vi "Queue Out.vi"(8 "error in (no error)":errorcluster caption="Error In", 10 "Monitor":string, 11 "Queue In":refnum<queue>) -> (0 "error out":errorcluster caption="Error Out", 1 "Data":variant, 2 "Message":string, 3 "Queue Out":refnum<queue>, 4 "Queue NUmber":i32)   [LabVIEW 2020]
uses:
  Queue Message.ctl
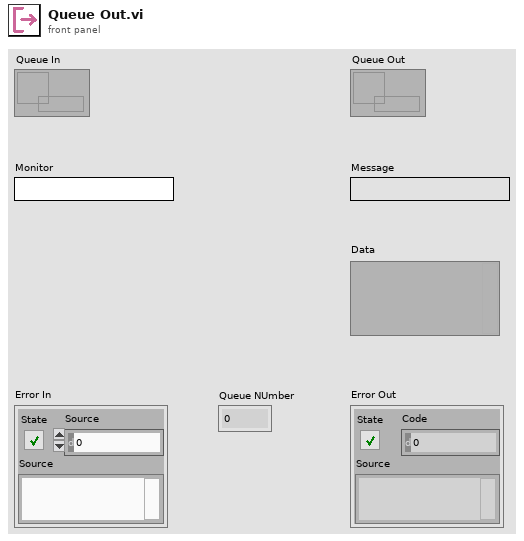
[diagram p1: front panel]
types:
  T1 = typedef "Queue Message.ctl" = cluster{"Message":string, "Data":variant}
  T2 = cluster{"Time":string, "Name":string, "Message":string, "Data":variant, "elements":i32}
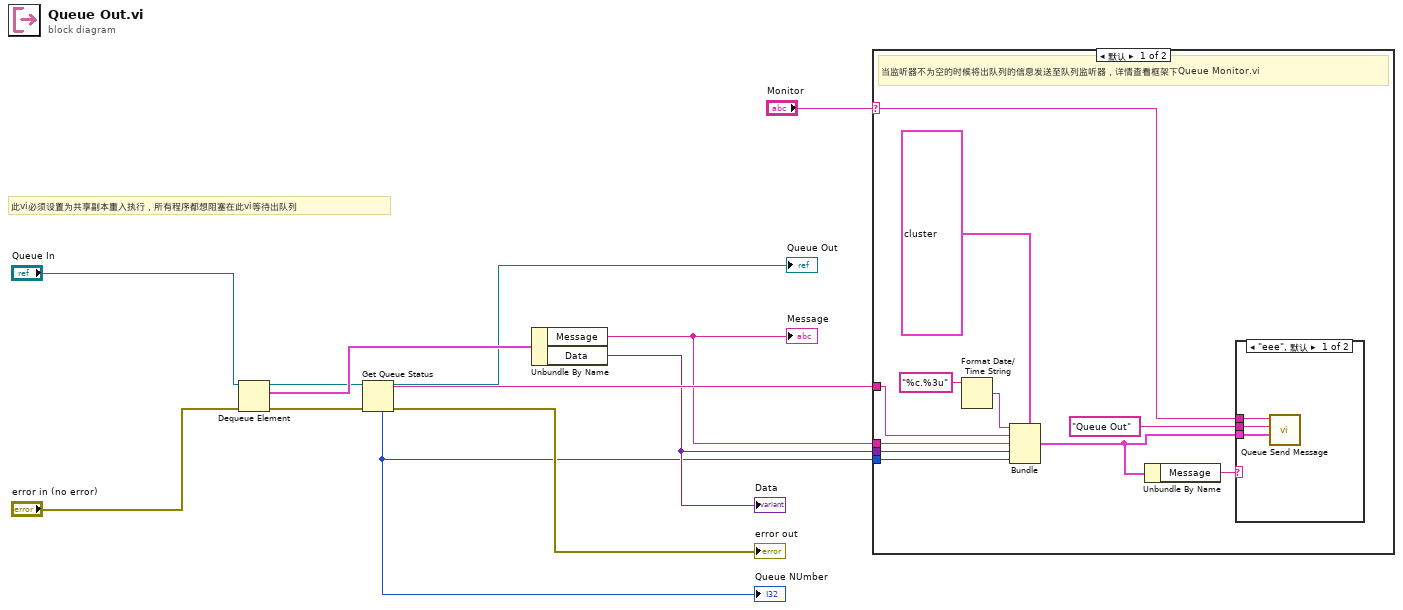
[diagram p0: block diagram]
diagram:
  # "此vi必须设置为共享副本重入执行，所有程序都想阻塞在此vi等待出队列"
  n1 = Dequeue Element(queue="Queue In", error in (no error)="error in (no error)") -> (queue out=w9:refnum<queue>, element=w11:T1, error out=w8:errorcluster)  [unwired: 1 in, 1 out]
  n2 = Get Queue Status(queue=w9, error in (no error)=w8) -> (queue out=→"Queue Out":refnum<queue>, queue name=w4:string, error out=→"error out":errorcluster, # elements in queue=w1:i32)  [unwired: 1 in, 4 out]
  "Queue NUmber" <- w1
  n3 = Unbundle By Name(w11) -> ("Message"=w3:string, "Data"=w2:variant)
  "Message" <- w3
  "Data" <- w2
  n4 = case shown="默认" "Monitor" {
    selector: "Monitor" -> [w23 _]
    tunnel: w4 -> [w20 _]
    tunnel: w3 -> [w19 _]
    tunnel: w2 -> [w18 _]
    tunnel: w1 -> [w17 _]
    frame Default {
      # "当监听器不为空的时候将出队列的信息发送至队列监听器，详情查看框架下Queue Monitor.vi"
      n5 = Format Date/Time String(time format string (%c)="%c.%3u" ("时间格式字符串(%c)")) -> (date/time string=w14:string)  [unwired: 2 in]
      n6 = Bundle(cluster=T2 {"Time"="", "Name"="", "Message"="", "Data"=variant, "elements"=0} ("Menu"), "Time"=w14, "Name"=w20, "Message"=w19, "Data"=w18, "elements"=w17) -> (w16:T2)
      n7 = Unbundle By Name(w16) -> ("Message"=w21:string)
      n8 = case shown="\"eee\", 默认" w21 {
        tunnel: w23 -> [w26 _]
        tunnel: "Queue Out" ("Message") -> [w25 _]
        tunnel: w16 -> [w24 _]
        frame "eee", Default {
          n9 = call "Queue Send Message.vi"("Data"=w24, "Message"=w25, "Queue Name"=w26) -> ()  [unwired: 6 in, 3 out]
        }
        frame "" {
        }
      }
    }
    frame "" {
    }
  }
